vi "Initialize Measurement Interface.vi"(8 "error in (no error)":errorcluster, 11 "niRFSTS Sequence Flow in":refnum<class "niRFSTS Sequence Flow.lvclass">) -> (0 "error out":errorcluster, 3 "niRFSTS Sequence Flow out":refnum<class "niRFSTS Sequence Flow.lvclass">)   [LabVIEW 2018, in "niRFSTS Sequence Flow.lvclass"]
uses:
  niRFSTS Sequence Flow.lvclass
  Plugins/Measurement Interface.lvlibp/Measurement Interface.lvclass
  niRFSTS Sequence Flow.lvclass/niRFSTS Sequence Flow.ctl
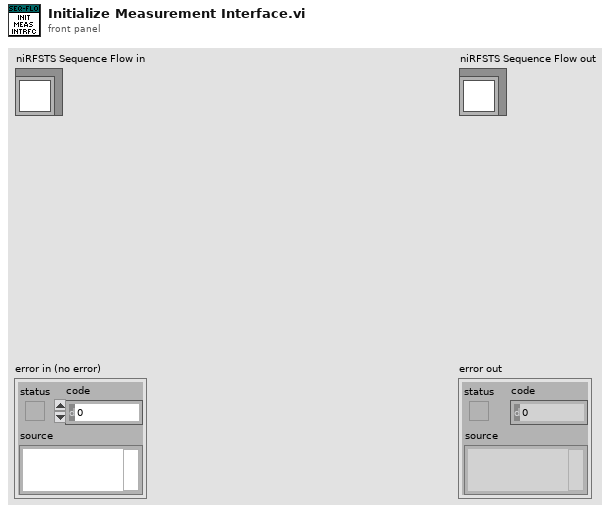
[diagram p1: front panel]
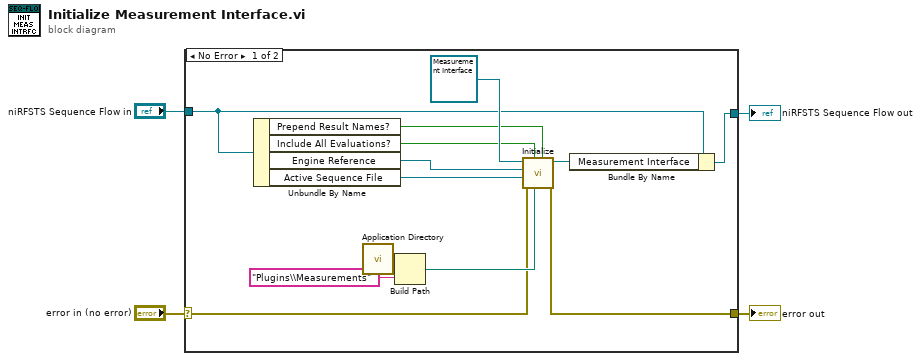
[diagram p0: block diagram]
diagram:
  n1 = case shown="No Error" "error in (no error)" {
    selector: "error in (no error)" -> [w10 w19]
    tunnel: [w9 w19] -> w3
    tunnel: [w8 w18] -> w1
    tunnel: "niRFSTS Sequence Flow in" -> [w13 w18]
    frame No Error {
      n2 = Unbundle By Name(w13) -> ("Prepend Result Names?"=w5:bool, "Include All Evaluations?"=w6:bool, "Engine Reference"=w12:refnum<k7>, "Active Sequence File"=w11:refnum<k7>)
      n3 = call <vilib>:"Application Directory.vi"() -> ("Application Directory"=w15:path)
      n4 = Build Path(base path=w15, name or relative path="Plugins\\Measurements") -> (appended path=w14:path)
      n5 = call-dynamic "Initialize.vi"("Prepend Result Name"=w5, "Folder Path"=w14, "Include All Evaluations?"=w6, "Error In"=w10, "Active Sequence File"=w11, "Engine Reference"=w12, "Measurement Interface In"=refnum<class "Measurement Interface.lvclass"> refnum ("Measurement Interface")) -> ("Error Out"=w9:errorcluster, "Measurement Interface out"=w7:refnum<class "Measurement Interface.lvclass">)  [unwired: 3 in]
      n6 = Bundle By Name(cluster=w13, "Measurement Interface"=w7) -> (w8:refnum<class "niRFSTS Sequence Flow.lvclass">)
    }
    frame Error {
    }
  }
  "error out" <- w3
  "niRFSTS Sequence Flow out" <- w1
